vi "get_exe_path.vi"() -> (0 "top level VI or exe":path, 1 "directory path":path, 2 "application root path":path, 3 "full path":path)   [LabVIEW 2020]
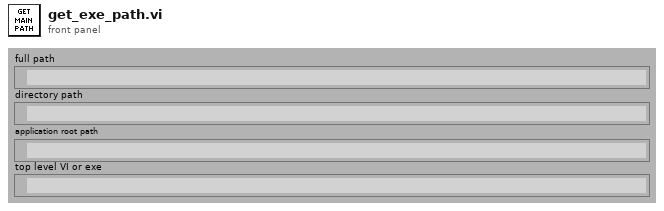
[diagram p1: front panel]
types:
  T1 = enum32{"invalid app kind", "Development System", "Run Time System", "Student Edition", "Embedded LabVIEW", "Evaluation", "Custom"}
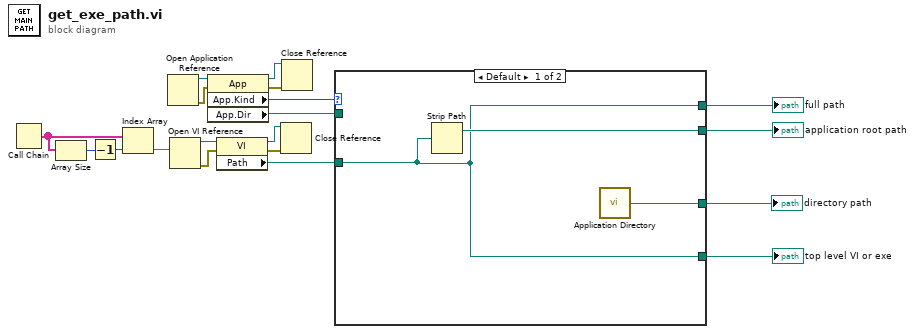
[diagram p0: block diagram]
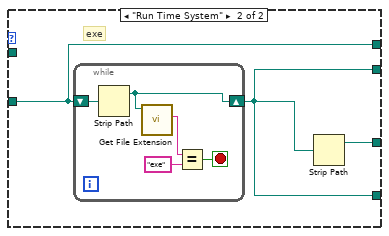
[diagram p2: hidden frame]
diagram:
  n1 = Call Chain() -> (call chain=w13:string[])
  n2 = Array Size(array=w13) -> (size(s)=w14:i32)
  n3 = Decrement(x=w14) -> (x-1=w12:i32)
  n4 = Index Array(array=w13, index=w12) -> (element=w11:string)
  n5 = Open Application Reference() -> (0:w6:errorcluster, 3:w17:refnum<vi>)  [unwired: 4 in]
  n6 = Open VI Reference(vi path=w11) -> (vi reference=w18:refnum<vi>, error out=w19:errorcluster)  [unwired: 5 in]
  n7 = property class="App"(reference=w17, error in=w6) -> (reference out=w9:refnum<vi>, error out=w10:errorcluster, "App.Kind"=w16:T1, "App.Dir"=w4:path)
  n8 = property class="VI"(reference=w18, error in=w19) -> (reference out=w7:refnum<vi>, error out=w8:errorcluster, "Path"=w15:path)
  n9 = Close Reference(reference=w7, error in (no error)=w8) -> ()  [unwired: 1 out]
  n10 = Close Reference(reference=w9, error in (no error)=w10) -> ()  [unwired: 1 out]
  n11 = case shown="Default" w16 {
    tunnel: w15 -> [w21 w25]
    tunnel: [w22 w24] -> w5
    tunnel: w4 -> [_ _]
    tunnel: [w21 w25] -> w3
    tunnel: [w21 w24] -> w2
    tunnel: [w20 w23] -> w1
    frame Default {
      n12 = Strip Path(path=w21) -> (stripped path=w22:path)  [unwired: 1 out]
      n13 = call <vilib>:"Application Directory.vi"() -> ("Application Directory"=w20:path)
    }
    frame "Run Time System" {
      # "exe"
      n14 = while {
        shift-right: [w26] -> w24
        shift-left: w25 -> [w27]
        stop <- w28 stop-if-true
        n15 = Strip Path(path=w27) -> (stripped path=w26:path)  [unwired: 1 out]
        n16 = call <vilib>:"Get File Extension.vi"("file"=w26) -> ("lowercase file extension"=w30:string)  [unwired: 6 in, 4 out]
        n17 = Equal?(x=w30, y="exe") -> (x = y?=w28:bool)
      }
      n18 = Strip Path(path=w24) -> (stripped path=w23:path)  [unwired: 1 out]
    }
  }
  "full path" <- w3
  "directory path" <- w1
  "application root path" <- w5
  "top level VI or exe" <- w2
